vi "Get Category.vi"(8 "error in (no error)":errorcluster, 11 "configuration in":refnum<class "dds configuration.lvclass">) -> (0 "error out":errorcluster, 2 "Category":string, 3 "configuration out":refnum<class "dds configuration.lvclass">)   [LabVIEW 2020, in "DDS configuration.lvclass"]
uses:
  dds configuration.lvclass
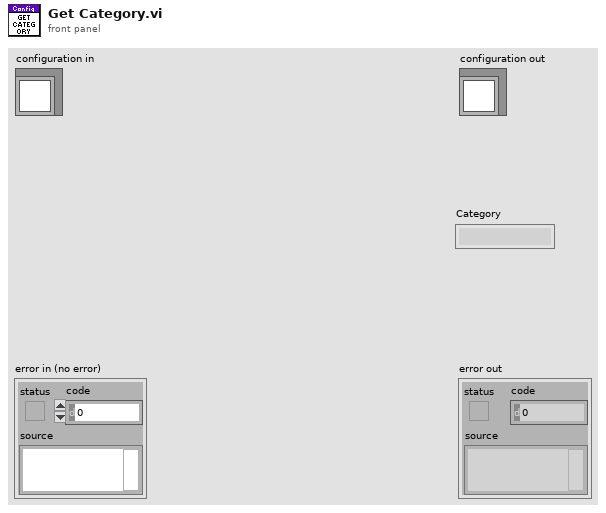
[diagram p1: front panel]
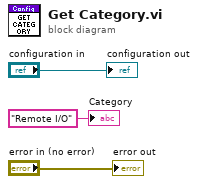
[diagram p0: block diagram]
diagram:
  "error out" <- "error in (no error)"
  "configuration out" <- "configuration in"
  "Category" <- "Remote I/O" ("Category")
